vi "Velox_ReadChuckPosition.vi"(8 "error in (no error)":errorcluster, 11 "VeloxTeslaProbestation in":refnum<class "VeloxTeslaProbestation.lvclass">) -> (0 "error out":errorcluster, 3 "VeloxTeslaProbestation out":refnum<class "VeloxTeslaProbestation.lvclass">)   [LabVIEW 2018, in "VeloxTeslaProbestation.lvclass"]
uses:
  VeloxTeslaProbestation.lvclass
  Desktop/Kvasnicka/test_labview_library/Integration_toolkit_library/CascadeProbestation.lvlib
panel:
  out "Response":string
  out "Z Value":dbl format="%.2f"
  out "Y Value":dbl format="%.2f"
  out "X Value":dbl format="%.2f"
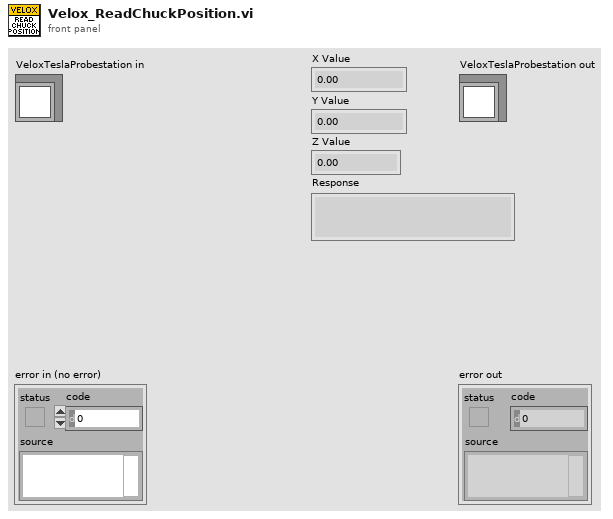
[diagram p1: front panel]
types:
  T1 = enum16{"Default", "Technology", "Offset", "Prober", "None"}
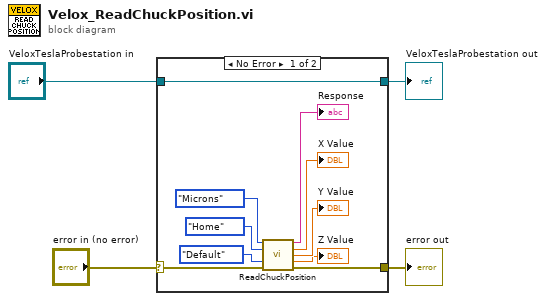
[diagram p0: block diagram]
diagram:
  n1 = case shown="No Error" "error in (no error)" {
    selector: "error in (no error)" -> [w7 w16]
    tunnel: [w6 w16] -> w3
    tunnel: [w14 w15] -> w1
    tunnel: "VeloxTeslaProbestation in" -> [w14 w15]
    frame No Error {
      n2 = call "ReadChuckPosition.vi"("Unit"=enum16{"Microns", "Mils", "Index"}."Microns", "PosRef"=enum16{"Home", "Zero", "Center"}."Home", "CompLevel"=T1."Default", "Error In"=w7) -> ("Response"=→"Response":string, "X Value"=→"X Value":dbl, "Y Value"=→"Y Value":dbl, "Z Value"=→"Z Value":dbl, "Error Out"=w6:errorcluster)  [unwired: 7 in]
    }
    frame Error {
    }
  }
  "error out" <- w3
  "VeloxTeslaProbestation out" <- w1
